vi "DelayPeriod.vi"(8 "error in (no error)":errorcluster, 11 "TrialBasedExperiment in":refnum<class "MatlabExperiment.lvclass">) -> (0 "error out":errorcluster, 2 "Timeout":dbl, 3 "TrialBasedExperiment out":refnum<class "MatlabExperiment.lvclass">)   [LabVIEW 2012, in "AcquisitionCoreObjects.lvlib" / "MatlabExperiment.lvclass"]
uses:
  MatlabExperiment.lvclass
  TrialBasedExperimentObject/TrialBasedExperiment.lvclass
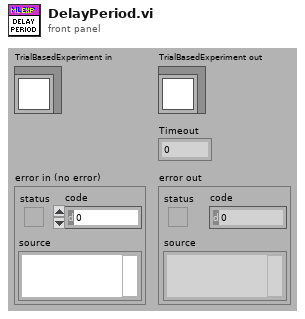
[diagram p1: front panel]
types:
  T1 = enum16{"StartSession", "StartTrial", "ShowStimulus"}
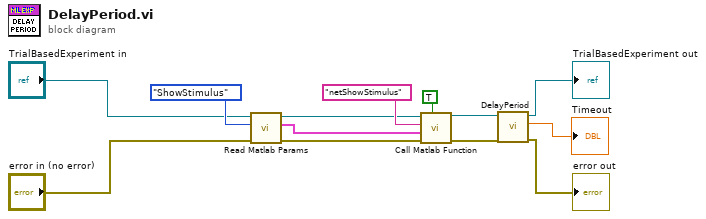
[diagram p0: block diagram]
diagram:
  n1 = call-dynamic "Read Matlab Params.vi"("error in (no error)"="error in (no error)", "Enum"=T1."ShowStimulus", "TrialBasedExperiment in"="TrialBasedExperiment in") -> ("error out"=w2:errorcluster, "Matlab Param Array"=w1:cluster{"Name":string, "Data":variant}[], "TrialBasedExperiment out"=w4:refnum<class "MatlabExperiment.lvclass">)  [unwired: 6 in]
  n2 = call-dynamic "Call Matlab Function.vi"("Timestamp"=TRUE, "error in (no error)"=w2, "Matlab Param Array"=w1, "Function name"="netShowStimulus", "TrialBasedExperiment in"=w4) -> ("error out"=w8:errorcluster, "TrialBasedExperiment out"=w7:refnum<class "MatlabExperiment.lvclass">)  [unwired: 3 in, 2 out]
  n3 = call-parent "DelayPeriod.vi"("error in (no error)"=w8, "TrialBasedExperiment in"=w7) -> ("error out"=→"error out":errorcluster, "Timeout"=→"Timeout":dbl, "TrialBasedExperiment out"=→"TrialBasedExperiment out":refnum<class "MatlabExperiment.lvclass">)  [unwired: 7 in]
